vi "Fail_Clock_2.vi"(11 "fail":i32) -> (8 "Trigger":dbl)   [LabVIEW 2017]
uses:
  BERTTA.dll
panel:
  out "TimeChange":dbl
  out "Elapsed":dbl
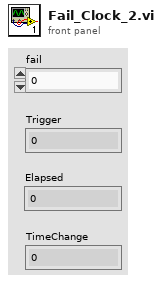
[diagram p1: front panel]
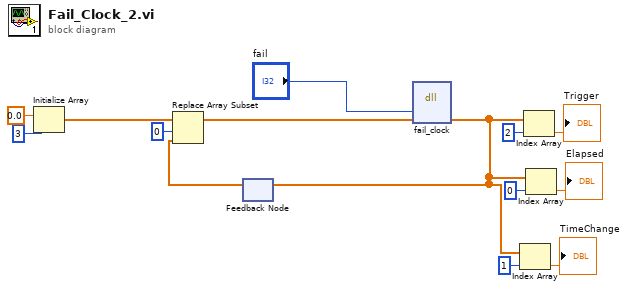
[diagram p0: block diagram]
diagram:
  n1 = Initialize Array(0.0 ("element"), 3 ("dimension size")) -> (w11:dbl[])
  n2 = feedback #1() -> (w14:dbl[])  [unwired: 1 in]
  n3 = Replace Array Subset(array=w11, new element=w14, index=0) -> (w12:dbl[])
  n4 = dll-call lib="C:/Users/shresplab/OneDrive - Kemira Oyj/Documents/GitHub/Bertta/BERTTA/x64/Debug/BERTTA.dll" fn="fail_clock"("fail"="fail", "params"=w12) -> ("params"=w1:dbl[])  [unwired: 5 in, 2 out]
  n5 = feedback-in #1(w1) -> ()
  n6 = Index Array(array=w1, index=1) -> (element=→"TimeChange":dbl)
  n7 = Index Array(array=w1, index=2) -> (element=→"Trigger":dbl)
  n8 = Index Array(array=w1, index=0) -> (element=→"Elapsed":dbl)
